vi "Condition.vi"(7 "_Rescript in":refnum<class "_Rescript.lvclass">, 8 "error in":errorcluster) -> (0 "error out":errorcluster, 5 "_Rescript out":refnum<class "_Rescript.lvclass">)   [LabVIEW 2025, in "_Rescript.lvlib" / "Msg.lvlib"]
uses:
  Msg.lvlib
  _Shared/Name Specs/Name Specs.lvclass
  _Rescript/_Rescript.lvclass
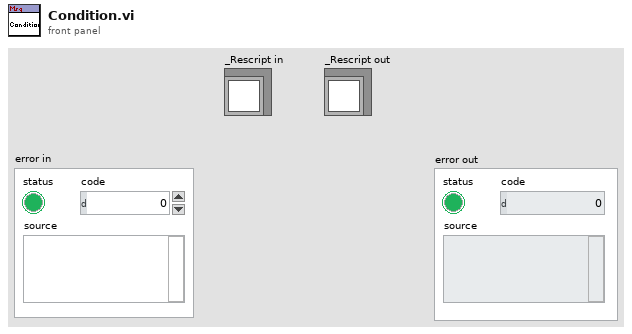
[diagram p1: front panel]
types:
  T1 = typedef "_Shared.lvlib/Name Stuff.ctl" = cluster{"Type (Enum)":T2, "Type (String)":string, "Name Library File Path":path, "Name":string, "Name Type":string}
  T2 = typedef "_Shared.lvlib/Type.ctl" = enum16{"Actor", "Msg"}
  T3 = typedef "_Rescript.lvlib/Terminal Attributes.ctl" = map{i32, T4}
  T4 = typedef "_Rescript.lvlib/Attributes.ctl" = cluster{"Control":refnum<vi>, "Wire Rule":enum16{"Invalid Wire Rule", "Required", "Recommended", "Optional", "Dynamic Dispatch"}}
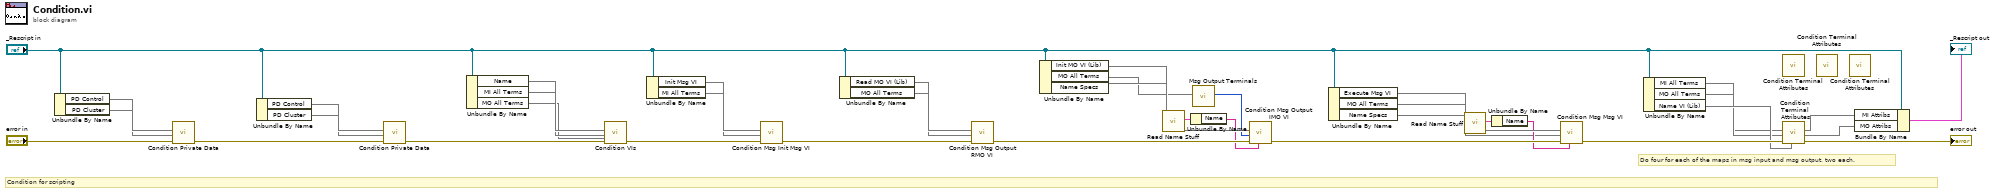
[diagram p0: block diagram]
diagram:
  # "Do four for each of the maps in msg input and msg output, two each."
  # "Condition for scripting"
  n1 = Unbundle By Name("_Rescript in") -> ("PD Control"=w37, "PD Cluster"=w36)
  n2 = call "Condition Private Data.vi"("error in"="error in", "Private Data Cluster"=w36, "Private Data Control"=w37) -> ("error out"=w30:errorcluster)  [unwired: 8 in]
  n3 = Unbundle By Name("_Rescript in") -> ("PD Control"=w28, "PD Cluster"=w27)
  n4 = call "Condition Private Data.vi"("error in"=w30, "Private Data Cluster"=w27, "Private Data Control"=w28) -> ("error out"=w29:errorcluster)  [unwired: 8 in]
  n5 = Unbundle By Name("_Rescript in") -> ("Name"=w31, "MI All Terms"=w26, "MO All Terms"=w22)
  n6 = call "Condition VIs.vi"("Msg Output All Terminals"=w22, "error in"=w29, "Msg All Terminals"=w26, "VI Refs"=w31) -> ("error out"=w32:errorcluster)  [unwired: 7 in]
  n7 = Unbundle By Name("_Rescript in") -> ("Init Msg VI"=w34, "MI All Terms"=w33)
  n8 = call "Condition Msg Init Msg VI.vi"("error in"=w32, "Msg All Terminals"=w33, "Name Msg Refs.Init Msg VI"=w34) -> ("error out"=w25:errorcluster)  [unwired: 8 in]
  n9 = Unbundle By Name("_Rescript in") -> ("Read MO VI (Lib)"=w21, "MO All Terms"=w20)
  n10 = call "Condition Msg Output RMO VI.vi"("error in"=w25, "Msg Output All Terminals"=w20, "Name Msg Output Refs.Read Msg Output VI"=w21) -> ("error out"=w24:errorcluster)  [unwired: 8 in]
  n11 = Unbundle By Name("_Rescript in") -> ("Init MO VI (Lib)"=w19, "MO All Terms"=w6, "Name Specs"=w18)
  n12 = call "Read Name Stuff.vi"("Name Specs in"=w18) -> ("Name Stuff"=w17:T1)  [unwired: 10 in]
  n13 = Unbundle By Name(w17) -> ("Name"=w16:string)
  n14 = call "Msg Output Terminals.vi"("Msg Output Terminals"=w6) -> ("Init Msg Output Terminals"=w5:i32[])  [unwired: 9 in, 1 out]
  n15 = call "Condition Msg Output IMO VI.vi"("Name"=w16, "error in"=w24, "Msg Output All Terminals (For Init Msg Output.vi)"=w5, "Name Msg Output Refs.Init Msg Output VI"=w19) -> ("error out"=w23:errorcluster)  [unwired: 7 in]
  n16 = Unbundle By Name("_Rescript in") -> ("Execute Msg VI"=w35, "MO All Terms"=w7, "Name Specs"=w9)
  n17 = call "Read Name Stuff.vi"("Name Specs in"=w9) -> ("Name Stuff"=w10:T1)  [unwired: 10 in]
  n18 = Unbundle By Name(w10) -> ("Name"=w8:string)
  n19 = call "Condition Msg Msg VI.vi"("Name"=w8, "error in"=w23, "Msg Output All Terminals"=w7, "Name Msg Refs.Msg VI"=w35) -> ("error out"=w38:errorcluster)  [unwired: 7 in]
  n20 = Unbundle By Name("_Rescript in") -> ("MI All Terms"=w11, "MO All Terms"=w12, "Name VI (Lib)"=w13)
  n21 = call "Condition Terminal Attributes.vi"() -> ()  [unwired: 10 in, 2 out]
  n22 = call "Condition Terminal Attributes.vi"(6:w13, "error in"=w38, "VI"=w12, "Terminals"=w11) -> ("error out"=→"error out":errorcluster, 1:w14, "Terminal Attributes"=w15:T3)  [unwired: 5 in]
  n23 = call "Condition Terminal Attributes.vi"() -> ()  [unwired: 10 in, 2 out]
  n24 = call "Condition Terminal Attributes.vi"() -> ()  [unwired: 10 in, 2 out]
  n25 = Bundle By Name(cluster="_Rescript in", "MI Attribs"=w15, "MO Attribs"=w14) -> (→"_Rescript out":cluster{})
